vi "SerialConnect.vi"(3 "error in (no error)":errorcluster, 4 "baud rate (9600)":u32=9600, 5 "VISA resource name":refnum<visa-resource-name>="COM1") -> (0 "error out":errorcluster)   [LabVIEW 2010]
uses:
  <vilib>/Instr/_visa.llb/VISA Configure Serial Port (Instr).vi
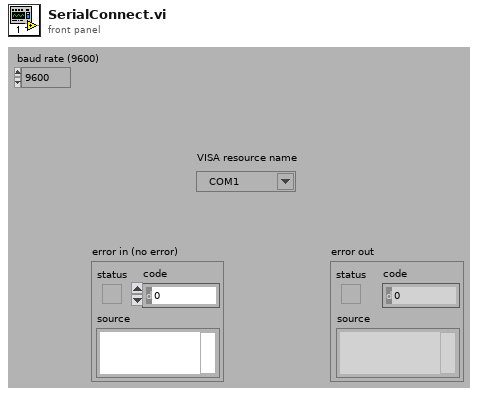
[diagram p1: front panel]
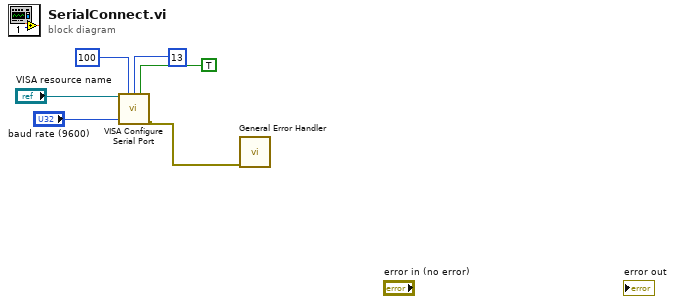
[diagram p0: block diagram]
diagram:
  n1 = call-poly "VISA Configure Serial Port"("VISA resource name"="VISA resource name", "timeout (10sec)"=u32 100, "termination char\n(0xA = '\\n' = LF)"=u8 13 ("termination char\n(0xA = '\\n' = LF)"), "Enable Termination\nChar (T)"=TRUE, "baud rate (9600)"="baud rate (9600)") -> ("error out"=w5:errorcluster)  [unwired: 9 in, 1 out]
  n2 = call <vilib>:"General Error Handler.vi"("error in (no error)"=w5) -> ()  [unwired: 1 in, 14 out]
